vi "From String.vi"(8 "error in (no error)":errorcluster, 9 "initial scan location":u32, 10 "String":string, 11 "Double Float in":refnum<class "Abs_Single Float.lvclass">) -> (0 "error out":errorcluster, 1 "offset past scan":u32, 2 "Remaining String":string, 3 "Double Float out":refnum<class "Abs_Single Float.lvclass">)   [LabVIEW 2021, in "Abs_Single Float.lvclass"]
uses:
  Abs_Single Float.lvclass
  C:/Program Files (x86)/National Instruments/LabVIEW 2021/vi.lib/TSA/Abstract Data Classes/Abs_Types/Numeric/Abs_Numeric.lvclass
  Support/Type.ctl
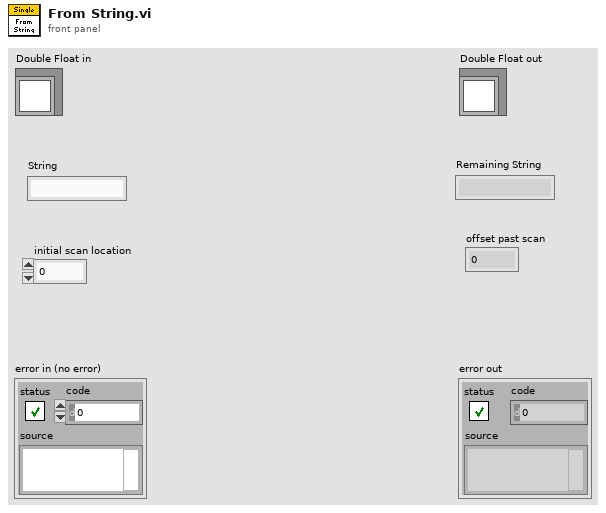
[diagram p1: front panel]
types:
  T1 = typedef "Abs_Single Float.lvclass/Type.ctl" = sgl
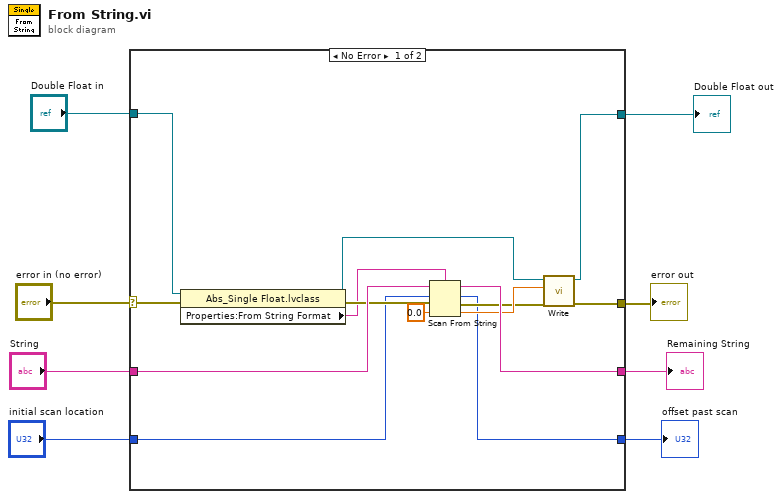
[diagram p0: block diagram]
diagram:
  n1 = case shown="No Error" "error in (no error)" {
    selector: "error in (no error)" -> [w17 w25]
    tunnel: [w22 w25] -> w8
    tunnel: "String" -> [w21 w24]
    tunnel: [w20 w24] -> w6
    tunnel: "Double Float in" -> [w15 w26]
    tunnel: [w11 w26] -> w3
    tunnel: "initial scan location" -> [w10 w23]
    tunnel: [w9 w23] -> w1
    frame No Error {
      n2 = property class="Abs_Single Float.lvclass"(reference=w15, error in=w17) -> (reference out=w12:refnum<class "Abs_Single Float.lvclass">, error out=w16:errorcluster, "Properties:From String Format"=w14:string)
      n3 = Scan From String(format string=w14, input string=w21, initial scan location=w10, error in=w16, default 1=T1 0.0 ("default value 1")) -> (remaining string=w20:string, offset past scan=w9:u32, error out=w18:errorcluster, output 1=w19:T1)
      n4 = call-dynamic "Write.vi"("error in (no error)"=w18, "Value"=w19, "Double Float.lvclass_340760 in"=w12) -> ("error out"=w22:errorcluster, "Double Float.lvclass_340760 out"=w11:refnum<class "Abs_Single Float.lvclass">)  [unwired: 7 in]
    }
    frame Error {
    }
  }
  "error out" <- w8
  "Double Float out" <- w3
  "Remaining String" <- w6
  "offset past scan" <- w1
